vi "emi_Tabs Grey out.vi"(0 "Tab Control":refnum<vi>, 7 "Tabs to Grey out":i32[](array[numeric]), 11 "error in":errorcluster) -> (4 "Tab Control out":refnum<vi>, 15 "error out":errorcluster)   [LabVIEW 2010]
doc: "Setting tab gray state based on an array of indexes.\n\nOn error: do nothing."
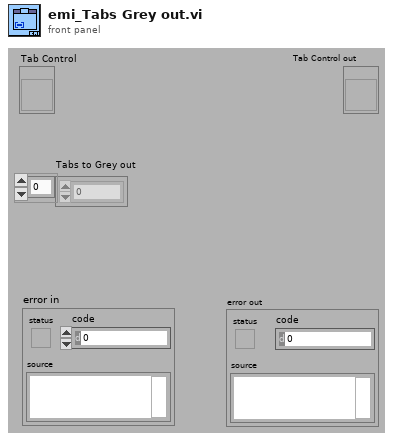
[diagram p1: front panel]
types:
  T1 = enum32{"Page Enabled", "Page Disabled", "Page Disabled & Grayed"}
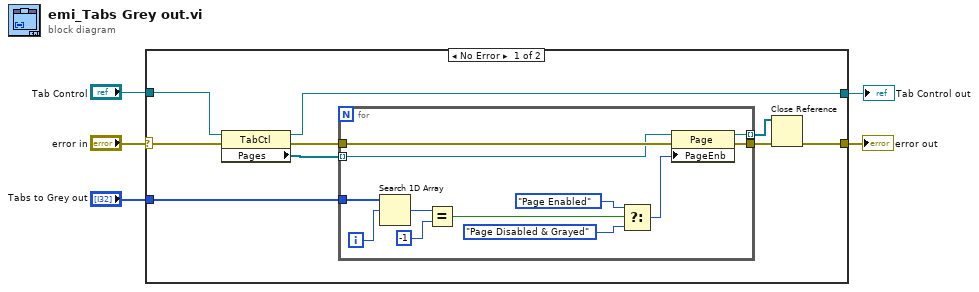
[diagram p0: block diagram]
diagram:
  n1 = case shown="No Error" "error in" {
    selector: "error in" -> [w7 w28]
    tunnel: "Tab Control" -> [w13 w27]
    tunnel: [w12 w27] -> w4
    tunnel: [w10 w28] -> w3
    tunnel: "Tabs to Grey out" -> [w6 _]
    frame No Error {
      n2 = property class="TabCtl"(reference=w13, error in=w7) -> (reference out=w12:refnum<vi>, error out=w14:errorcluster, "Pages"=w11:refnum<vi>[])
      n3 = for {
        tunnel: w14 -> [w26]
        tunnel: [w25] -> w9
        tunnel: w11 -> [w24] mode=indexing
        tunnel: [w23] -> w8 mode=indexing
        tunnel: w6 -> [w22]
        i -> [w21]
        n4 = Search 1D Array(1D array=w22, element=w21) -> (index of element=w20:i32)  [unwired: 1 in]
        n5 = Equal?(x=w20, y=-1) -> (x = y?=w18:bool)
        n6 = Select(t=T1."Page Enabled" ("Page Enabled State"), s=w18, f=T1."Page Disabled & Grayed" ("Page Enabled State")) -> (s? t:f=w15:T1)
        n7 = property class="Page"(reference=w24, error in=w26, "PageEnb"=w15) -> (reference out=w23:refnum<vi>, error out=w25:errorcluster)
      }
      n8 = Close Reference(reference=w8, error in (no error)=w9) -> (error out=w10:errorcluster)
    }
    frame Error {
    }
  }
  "error out" <- w3
  "Tab Control out" <- w4
